vi "Event Handler.vi"(0 "uService Template in":refnum<class "Common GUI v3.lvclass">, 5 "Event type":T1=enum."Message", 7 "Item Name":string, 9 "Data":variant, 11 "error in (no error)":errorcluster) -> (4 "uService Template out":refnum<class "Common GUI v3.lvclass">, 15 "error out":errorcluster)   [LabVIEW 2026, in "TALOS.lvlib" / "Common GUI v3.lvlib" / "Common GUI v3.lvclass"]
uses:
  Common GUI v3.lvclass
  C:/LabVIEW Code/TALOS/talos/Father of all uServices/Father of all uServices/Father of all uServices.lvclass
  Father of all uServices/Father of all uServices/Event Handler Items.ctl
  Ancestor/Ancestor/Ancestor.lvclass/Ancestor.ctl
  Common GUI v3 Consumer Case Selector.ctl
  Father of all uServices/Father of all uServices Messages/Consumer Msg/Consumer Msg.lvclass/Consumer Msg.ctl
  Common GUI v3.lvclass/Common GUI v3.ctl
  FGV/Error Memory/Get Error Description.vi
  Support VIs/Get PC name.vi
  Ancestor/Ancestor/Read ID.vi
  Support VIs/Get Class Name.vi
  <vilib>/Utility/error.llb/Clear Errors.vi
  Father of all uServices/Father of all uServices Messages/Consumer Msg/Send Consumer.vi
  FGV/Error Memory/Error Memory Core.vi
  <vilib>/AdvancedString/Delimited String to 1D String Array.vi
  <vilib>/AdvancedString/Delimited String to 1D String Array (string).vi
  Support VIs/Circus Root Path.vi
  FGV/Error Memory/Error Crt Lvl checker.vi
  FGV/Error Memory/Error Memory Core.vi/40c8088d-b597-4017-91af-faa98e00292e.vi
  FGV/Error Memory/Error Memory Core.vi/d4a3ab98-063c-4e44-b43d-fbdcfe6c2be2.vi
  Father of all uServices/Father of all uServices/Father of all uServices.lvclass
  C:/LabVIEW Code/TALOS/builds/Actor Framework PPL/Actor Framework.lvlibp/1abvi3w/vi.lib/ActorFramework/Actor/Actor.lvclass
  Support VIs/Global Memory.vi
  <vilib>/Utility/LVClass/Get LV Class Name.vi
  Support VIs/Is in Packed Library.vi
  Support VIs/TALOS Root path.vi
  Support VIs/Read CSV worksheet.vi
  Support VIs/Global Constants.vi
  <vilib>/Utility/error.llb/General Error Handler.vi
  builds/Actor Framework PPL/Actor Framework.lvlibp/1abvi3w/vi.lib/ActorFramework/Actor/Read Self Enqueuer.vi
  <userlib>/_OpenG.lib/lvdata/lvdata.llb/Get Strings from Enum__ogtk.vi
  builds/Actor Framework PPL/Actor Framework.lvlibp/1abvi3w/vi.lib/ActorFramework/Message Enqueuer/Enqueue.vi
  Support VIs/Error Log.vi
  Ancestor/Ancestor/Ancestor.lvclass
  <vilib>/Comparison/Equal/Equal Functor/Equal Functor.lvclass
  Father of all uServices/Father of all uServices Messages/Consumer Msg/Consumer Msg.lvclass
  TALOS.lvlib
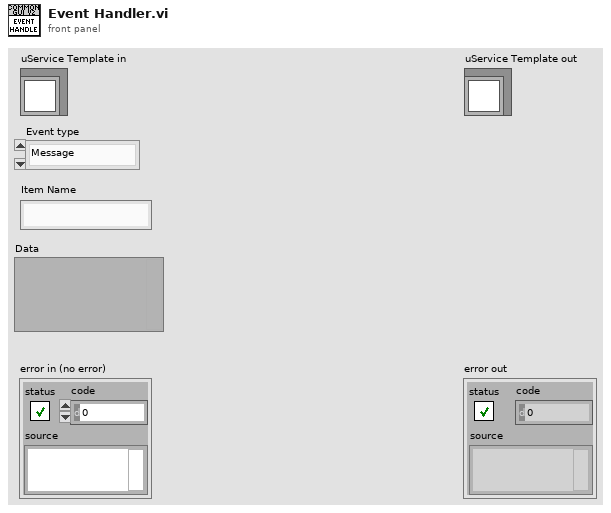
[diagram p1: front panel]
types:
  T1 = typedef "TALOS.lvlib/Father of all uServices.lvlib/Father of all uServices.lvclass/Event Handler Items.ctl" = enum16{"Button Pressed", "Message", "Ready to launch?", "Safe Mode", "Start RUN", "Stop RUN"}
  T2 = typedef "TALOS.lvlib/Common GUI v3.lvlib/Common GUI v3.lvclass/Common GUI v3 Consumer Case Selector.ctl" = enum16{"Update Guardians List", "Update ABORT LED", "Update Guardian ID", "Update Kasli Log", "Update Error Listbox", "Update Run Number", "Change Run LED color", "Update Run Status", "Run Stopped with Errors", "Reset Run LED", "Update Run Config", "Remote GUI"}
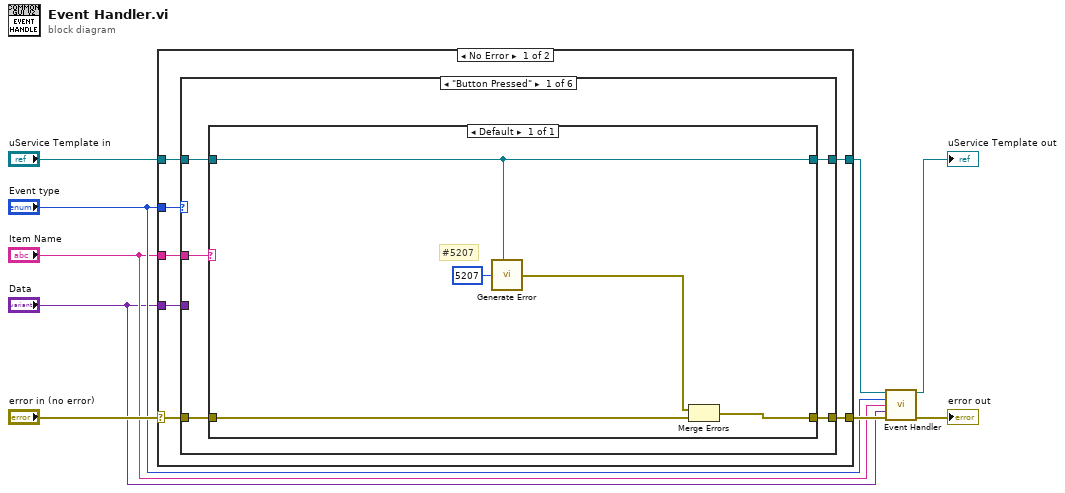
[diagram p0: block diagram]
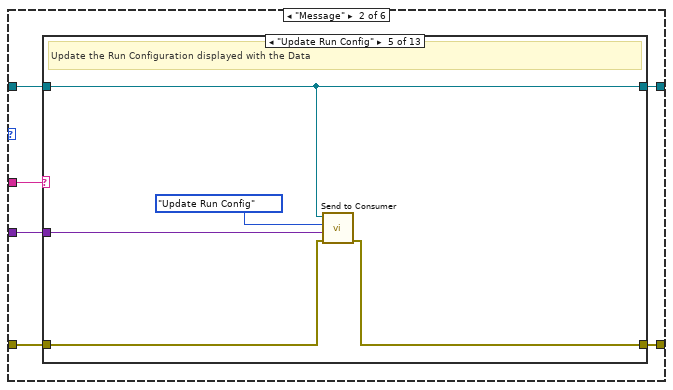
[diagram p2: hidden frame]
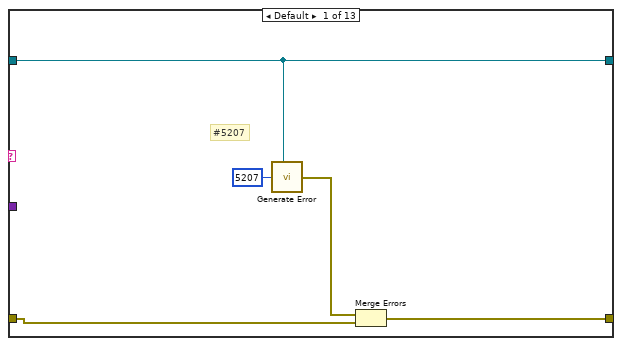
[diagram p3: hidden frame]
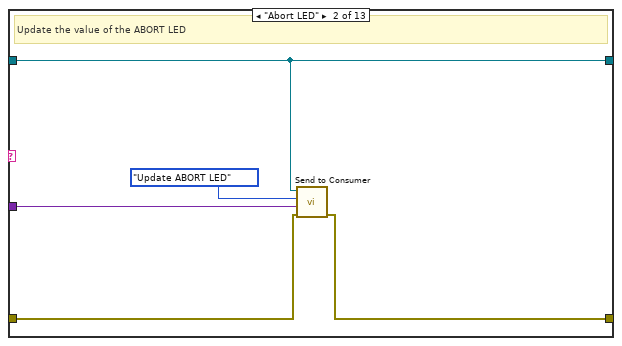
[diagram p4: hidden frame]
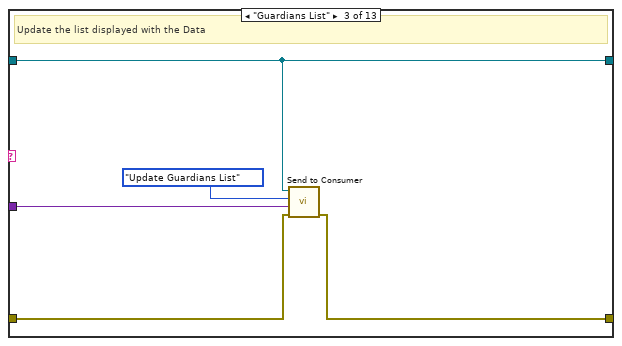
[diagram p5: hidden frame]
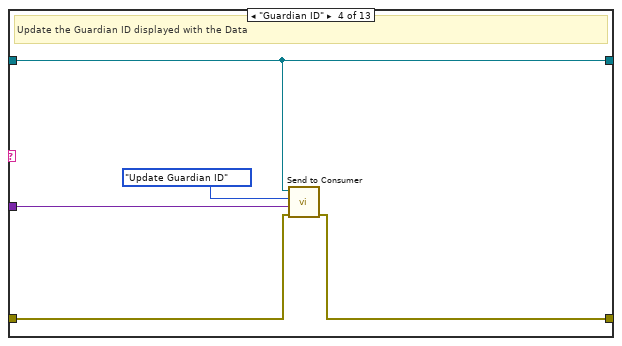
[diagram p6: hidden frame]
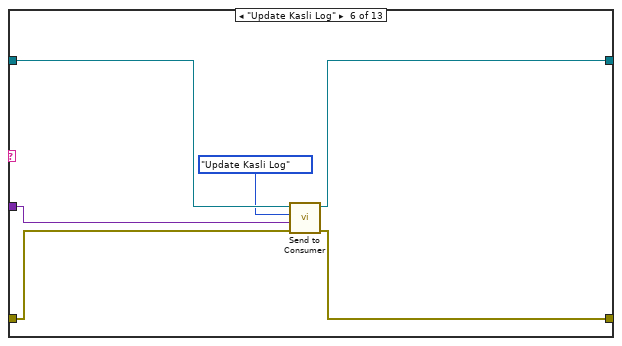
[diagram p7: hidden frame]
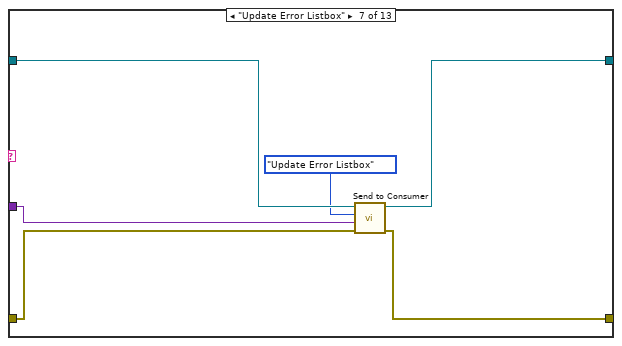
[diagram p8: hidden frame]
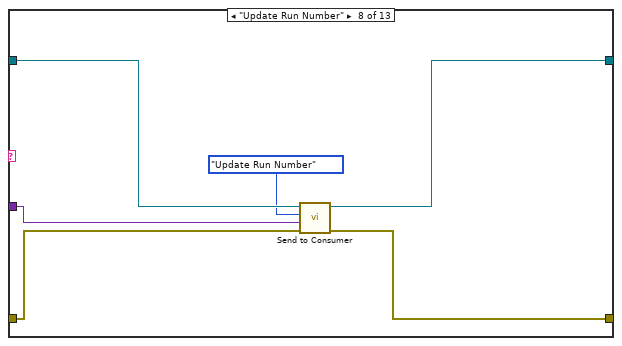
[diagram p9: hidden frame]
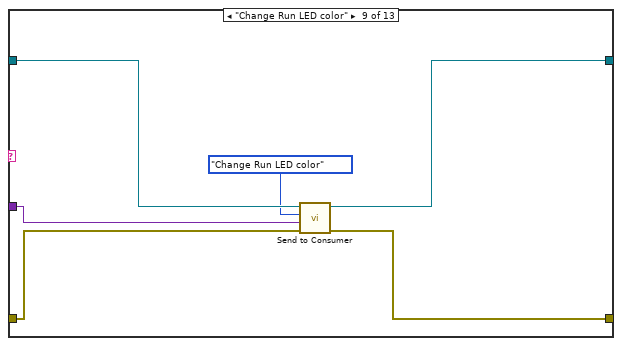
[diagram p10: hidden frame]
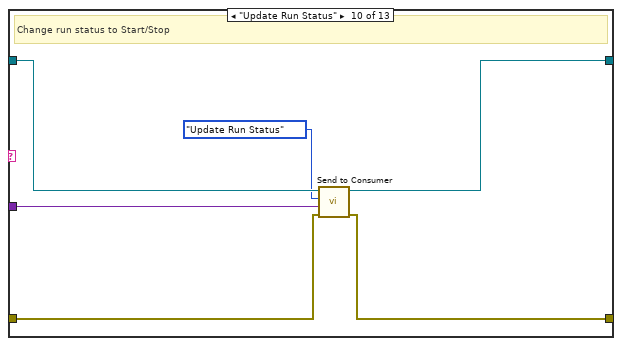
[diagram p11: hidden frame]
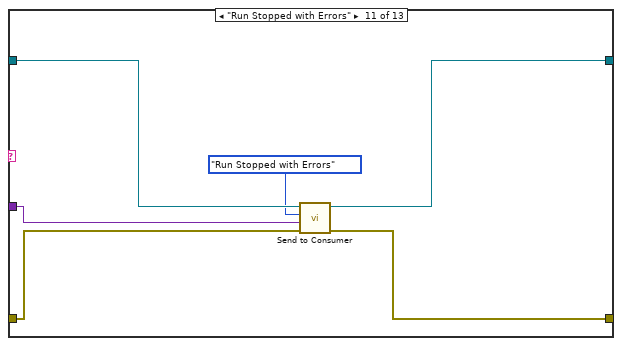
[diagram p12: hidden frame]
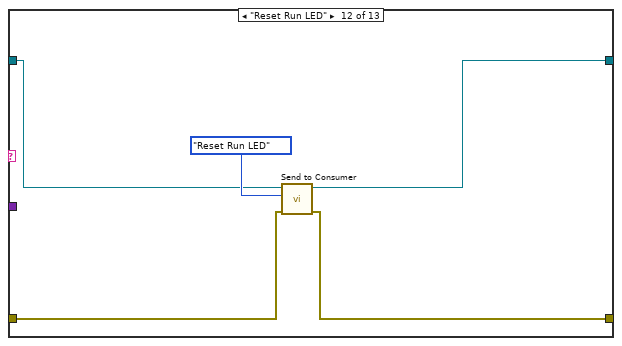
[diagram p13: hidden frame]
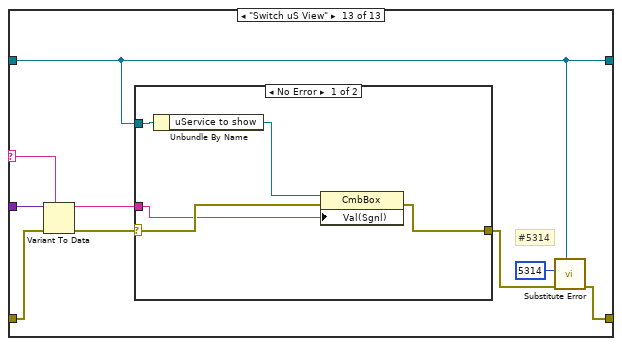
[diagram p14: hidden frame]
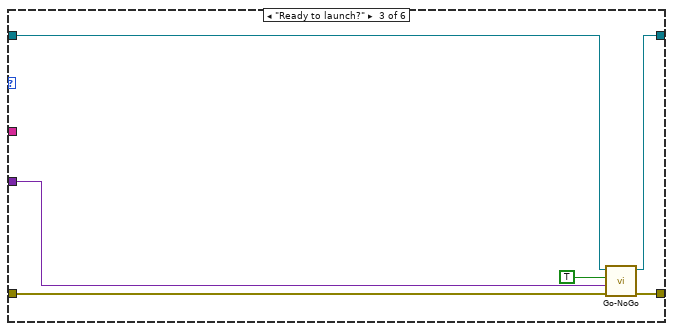
[diagram p16: hidden frame]
diagram:
  n1 = case shown="No Error" "error in (no error)" {
    selector: "error in (no error)" -> [w13 w127]
    tunnel: [w12 w127] -> w7
    tunnel: "uService Template in" -> [w15 w126]
    tunnel: [w14 w126] -> w4
    tunnel: "Event type" -> [w16 _]
    tunnel: "Item Name" -> [w11 _]
    tunnel: "Data" -> [w10 _]
    frame No Error {
      n2 = case shown="\"Button Pressed\"" w16 {
        tunnel: w15 -> [w21 w32 w116 w121 w122 w124]
        tunnel: [w20 w28 w119 w121 w122 w124] -> w14
        tunnel: w13 -> [w17 w29 w117 w120 w123 w125]
        tunnel: [w18 w27 w118 w120 w123 w125] -> w12
        tunnel: w11 -> [w19 w31 _ _ _ _]
        tunnel: w10 -> [_ w30 w114 _ _ _]
        frame "Button Pressed" {
          n3 = case shown="Default" w19 {
            tunnel: w21 -> [w22]
            tunnel: [w22] -> w20
            tunnel: [w25] -> w18
            tunnel: w17 -> [w26]
            frame Default {
              # "#5207"
              n4 = call "Generate Error.vi"("Class"=w22, "Error Code"=5207) -> ("error out"=w24:errorcluster)  [unwired: 5 in]
              n5 = Merge Errors(w24, w26) -> (w25:errorcluster)
            }
          }
        }
        frame "Message" {
          n6 = case shown="\"Update Run Config\"" w31 {
            selector: w31 -> [_ _ _ _ _ _ _ _ _ _ _ _ w106]
            tunnel: w32 -> [w35 w40 w45 w50 w55 w60 w66 w72 w78 w87 w90 w97 w100]
            tunnel: w30 -> [_ w41 w47 w52 w57 w63 w69 w75 w81 w83 w93 _ w107]
            tunnel: w29 -> [w33 w38 w43 w48 w53 w62 w68 w74 w80 w84 w92 w95 w105]
            tunnel: [w35 w40 w45 w50 w55 w59 w65 w71 w77 w86 w89 w96 w100] -> w28
            tunnel: [w34 w39 w44 w49 w54 w61 w67 w73 w79 w85 w91 w94 w101] -> w27
            frame Default {
              # "#5207"
              n7 = call "Generate Error.vi"("Class"=w35, "Error Code"=5207) -> ("error out"=w36:errorcluster)  [unwired: 5 in]
              n8 = Merge Errors(w36, w33) -> (w34:errorcluster)
            }
            frame "Abort LED" {
              # "Update the value of the ABORT LED"
              n9 = call "Send to Consumer.vi"("error in (no error)"=w38, "Data"=w41, "Case ID"=Common_GUI_v3_Consumer_Case_Selector."Update ABORT LED", "uService Template in"=w40) -> ("error out"=w39:errorcluster)  [unwired: 6 in, 1 out]
            }
            frame "Guardians List" {
              # "Update the list displayed with the Data"
              n10 = call "Send to Consumer.vi"("error in (no error)"=w43, "Data"=w47, "Case ID"=Common_GUI_v3_Consumer_Case_Selector."Update Guardians List", "uService Template in"=w45) -> ("error out"=w44:errorcluster)  [unwired: 6 in, 1 out]
            }
            frame "Guardian ID" {
              # "Update the Guardian ID displayed with the Data"
              n11 = call "Send to Consumer.vi"("error in (no error)"=w48, "Data"=w52, "Case ID"=Common_GUI_v3_Consumer_Case_Selector."Update Guardian ID", "uService Template in"=w50) -> ("error out"=w49:errorcluster)  [unwired: 6 in, 1 out]
            }
            frame "Update Run Config" {
              # "Update the Run Configuration displayed with the Data"
              n12 = call "Send to Consumer.vi"("error in (no error)"=w53, "Data"=w57, "Case ID"=Common_GUI_v3_Consumer_Case_Selector."Update Run Config", "uService Template in"=w55) -> ("error out"=w54:errorcluster)  [unwired: 6 in, 1 out]
            }
            frame "Update Kasli Log" {
              n13 = call "Send to Consumer.vi"("error in (no error)"=w62, "Data"=w63, "Case ID"=Common_GUI_v3_Consumer_Case_Selector."Update Kasli Log" ("Template Internal v3 Consumer Case Selector"), "uService Template in"=w60) -> ("error out"=w61:errorcluster, "uService Template out"=w59:refnum<class "Common GUI v3.lvclass">)  [unwired: 6 in]
            }
            frame "Update Error Listbox" {
              n14 = call "Send to Consumer.vi"("error in (no error)"=w68, "Data"=w69, "Case ID"=Common_GUI_v3_Consumer_Case_Selector."Update Error Listbox" ("Template Internal v3 Consumer Case Selector"), "uService Template in"=w66) -> ("error out"=w67:errorcluster, "uService Template out"=w65:refnum<class "Common GUI v3.lvclass">)  [unwired: 6 in]
            }
            frame "Update Run Number" {
              n15 = call "Send to Consumer.vi"("error in (no error)"=w74, "Data"=w75, "Case ID"=Common_GUI_v3_Consumer_Case_Selector."Update Run Number" ("Template Internal v3 Consumer Case Selector"), "uService Template in"=w72) -> ("error out"=w73:errorcluster, "uService Template out"=w71:refnum<class "Common GUI v3.lvclass">)  [unwired: 6 in]
            }
            frame "Change Run LED color" {
              n16 = call "Send to Consumer.vi"("error in (no error)"=w80, "Data"=w81, "Case ID"=Common_GUI_v3_Consumer_Case_Selector."Change Run LED color" ("Template Internal v3 Consumer Case Selector"), "uService Template in"=w78) -> ("error out"=w79:errorcluster, "uService Template out"=w77:refnum<class "Common GUI v3.lvclass">)  [unwired: 6 in]
            }
            frame "Update Run Status" {
              # "Change run status to Start/Stop"
              n17 = call "Send to Consumer.vi"("error in (no error)"=w84, "Data"=w83, "Case ID"=Common_GUI_v3_Consumer_Case_Selector."Update Run Status" ("Template Internal v3 Consumer Case Selector"), "uService Template in"=w87) -> ("error out"=w85:errorcluster, "uService Template out"=w86:refnum<class "Common GUI v3.lvclass">)  [unwired: 6 in]
            }
            frame "Run Stopped with Errors" {
              n18 = call "Send to Consumer.vi"("error in (no error)"=w92, "Data"=w93, "Case ID"=Common_GUI_v3_Consumer_Case_Selector."Run Stopped with Errors" ("Template Internal v3 Consumer Case Selector"), "uService Template in"=w90) -> ("error out"=w91:errorcluster, "uService Template out"=w89:refnum<class "Common GUI v3.lvclass">)  [unwired: 6 in]
            }
            frame "Reset Run LED" {
              n19 = call "Send to Consumer.vi"("error in (no error)"=w95, "Case ID"=Common_GUI_v3_Consumer_Case_Selector."Reset Run LED" ("Template Internal v3 Consumer Case Selector"), "uService Template in"=w97) -> ("error out"=w94:errorcluster, "uService Template out"=w96:refnum<class "Common GUI v3.lvclass">)  [unwired: 7 in]
            }
            frame "Switch uS View" {
              # "#5314"
              n20 = Variant To Data(error in=w105, type=w106, Variant=w107) -> (data=w103:string, error out=w104:errorcluster)
              n21 = case shown="No Error" w104 {
                selector: w104 -> [w110 w113]
                tunnel: w100 -> [w112 _]
                tunnel: w103 -> [w109 _]
                tunnel: [w108 w113] -> w102
                frame No Error {
                  n22 = Unbundle By Name(w112) -> ("uService to show"=w111:refnum<vi>)
                  n23 = property class="CmbBox"(reference=w111, error in=w110, "Val(Sgnl)"=w109) -> (error out=w108:errorcluster)  [unwired: 1 out]
                }
                frame Error {
                }
              }
              n24 = call "Substitute Error.vi"("LabVIEW Object"=w100, "error in (no error)"=w102, "Error Code"=5314) -> ("error out"=w101:errorcluster)  [unwired: 8 in]
            }
          }
        }
        frame "Ready to launch?" {
          n25 = call-dynamic "Go-NoGo.vi"("error in (no error)"=w117, "Go-NoGo Data"=w114, "Go?"=TRUE, "Father of all uServices in"=w116) -> ("error out"=w118:errorcluster, "Father of all uServices out"=w119:refnum<class "Common GUI v3.lvclass">)  [unwired: 6 in]
        }
        frame "Safe Mode" {
        }
        frame "Start RUN" {
        }
        frame "Stop RUN" {
        }
      }
    }
    frame Error {
    }
  }
  n26 = call-parent "Event Handler.vi"("uService Template in"=w4, "Event type"="Event type", "Item Name"="Item Name", "Data"="Data", "error in (no error)"=w7) -> ("uService Template out"=→"uService Template out":refnum<class "Common GUI v3.lvclass">, "error out"=→"error out":errorcluster)  [unwired: 9 in]
